vi "Parse TC Setups.vi"(3 "DB Data":string[][](array[string])) -> (1 "TC Parameters":T1)   [LabVIEW 2015, in "Config Data.lvlib" / "Config Data_DB_ADO.lvclass"]
uses:
  Config Data_DB_ADO.lvclass
  Startup Processes/_typedefs/TC Setup Parameters.ctl
  Startup Processes/Startup Processes.lvlib
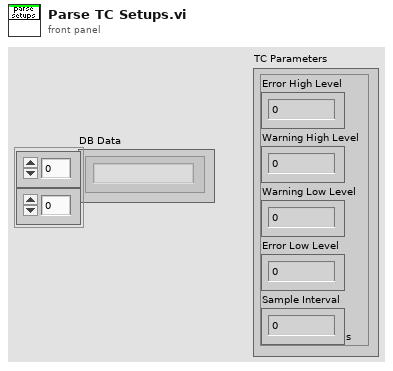
[diagram p1: front panel]
types:
  T1 = typedef "Startup Processes.lvlib/TC Setup Parameters.ctl" = cluster{"Error High Level":dbl, "Warning High Level":dbl, "Warning Low Level":dbl, "Error Low Level":dbl, "Sample Interval":dbl[unit]}
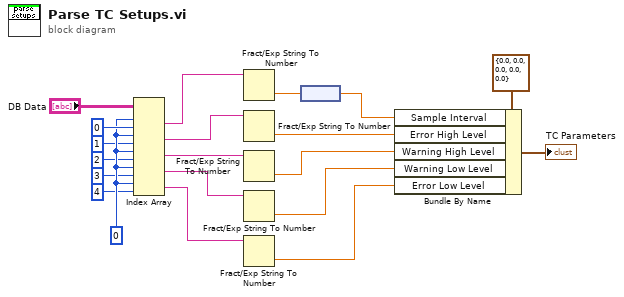
[diagram p0: block diagram]
diagram:
  w7 = 0 ("disabled index (col)")
  n1 = Index Array(array="DB Data", index (row) #1=w7, index (col) #1=0 ("disabled index (col)"), index (row) #2=w7, index (col) #2=1 ("disabled index (col)"), index (row) #3=w7, index (col) #3=2 ("disabled index (col)"), index (row) #4=w7, index (col) #4=3 ("disabled index (col)"), index (row) #5=w7, index (col) #5=4 ("disabled index (col)")) -> (element #1=w12:string, element #2=w11:string, element #3=w10:string, element #4=w9:string, element #5=w8:string)
  n2 = Fract/Exp String To Number(string=w12) -> (number=w14:dbl)  [unwired: 3 in, 1 out]
  n3 = Fract/Exp String To Number(string=w11) -> (number=w16:dbl)  [unwired: 3 in, 1 out]
  n4 = Fract/Exp String To Number(string=w10) -> (number=w17:dbl)  [unwired: 3 in, 1 out]
  n5 = Fract/Exp String To Number(string=w9) -> (number=w18:dbl)  [unwired: 3 in, 1 out]
  n6 = Fract/Exp String To Number(string=w8) -> (number=w19:dbl)  [unwired: 3 in, 1 out]
  n7 = node(w14) -> (w15:dbl[unit])
  n8 = Bundle By Name(cluster=T1 {"Error High Level"=0.0, "Warning High Level"=0.0, "Warning Low Level"=0.0, "Error Low Level"=0.0, "Sample Interval"=0.0} ("TC Parameters"), "Sample Interval"=w15, "Error High Level"=w16, "Warning High Level"=w17, "Warning Low Level"=w18, "Error Low Level"=w19) -> (→"TC Parameters":T1)
